vi "Create Table Refnum.vi"(0 "PDF Report":refnum<class "PDF Report Class.lvclass">, 1 "Table properties":T1={"Table position"=1, "SpacingBefore (points)"=12.0, "SpacingAfter (points)"=12.0} {"Table position" items=["LEFT", "CENTER", "RIGHT"]}, 5 "numColumns":i32, 9 "columnWidth [ ]":sgl[](array[numeric])=[0.0], 11 "error in (no error)":errorcluster, 12 "Repeat on each new page?":bool, 13 "HeaderRows":i32) -> (4 "PDF Report duplicate":refnum<class "PDF Report Class.lvclass">, 6 "columnWidth (points)":sgl[](array[numeric]), 8 "PdfP Table ref":refnum<k24>, 15 "error out":errorcluster)   [LabVIEW 2019]
doc: "<B>ENGLISH</B>\nCreates a table with the given <B>numColumns</B> and the given <B>columnWidth [ ]</B>.\n\n<B>FRANÇAIS</B>\nCréation d'un tableau avec pour nombre de colonnes <B>numColumns</B> et dont les largeurs sont spécifiées par <B>columnWidth [ ]</B>.\n\nVersion 2.0\nDeveloped by Jean-Marc Simard\nCopyright © 2012, Exaprom Inc.\nAll rights reserved.\nLicense: BSD\n\nWith iTextSharp 4.1.6 (http://itextsharp.sourceforge.net)\nunder Mozilla Public License Version 1.1\n(http://www.mozilla.org/MPL/MPL-1.1.html)"
uses:
  <userlib>/Exaprom PDF/LV Class/PDF Report Class/PDF Report Class.lvclass
  C:/Program Files/National Instruments/LabVIEW 2019/user.lib/Exaprom PDF/DLL/itextsharp.dll
  DLL/itextsharp.dll
  <userlib>/Exaprom PDF/Controls/Table Controls/Table properties.ctl
  <userlib>/Exaprom PDF/Controls/Table Controls/Table position.ctl
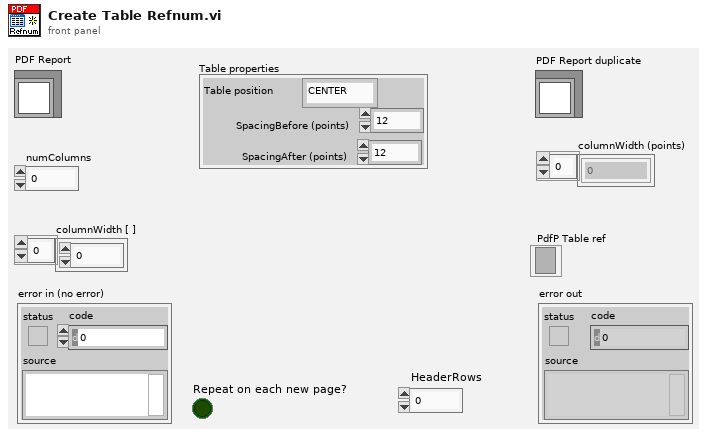
[diagram p1: front panel]
types:
  T1 = typedef "Table properties.ctl" = cluster{"Table position":T2, "SpacingBefore (points)":sgl, "SpacingAfter (points)":sgl}
  T2 = typedef "Table position.ctl" = i32
  T3 = typedef "Page dimensions.ctl" = cluster{"Start at page":i32, "Page Size":T4, "Orientation":T5, "widht":sgl, "height":sgl, "Margin left":sgl, "Margin right":sgl, "Margin top":sgl, "Margin bottom":sgl, "X0":sgl, "X1":sgl, "Y0":sgl, "Y1":sgl}
  T4 = typedef "Page size.ctl" = i32
  T5 = typedef "Page Orientation.ctl" = enum16{"Portrait", "Landscape"}
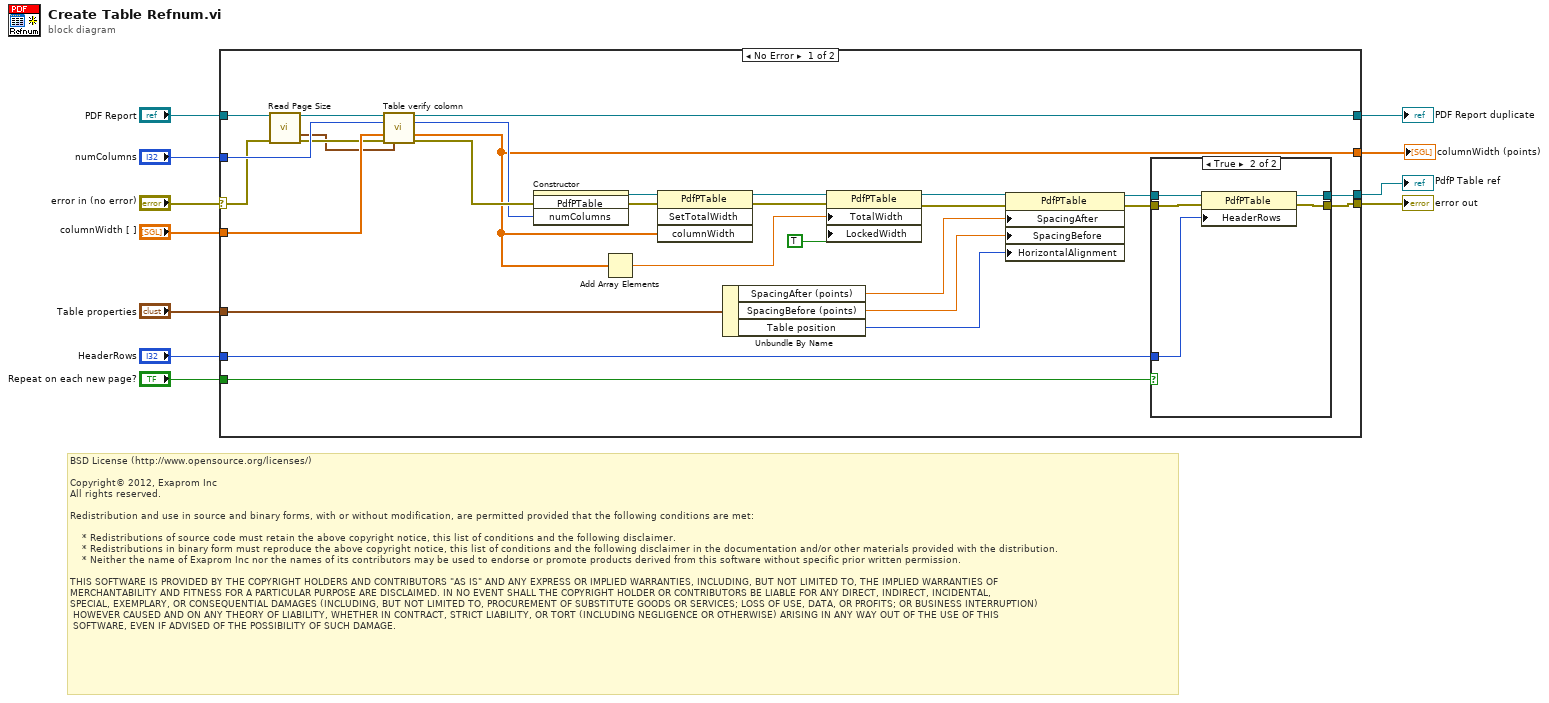
[diagram p0: block diagram]
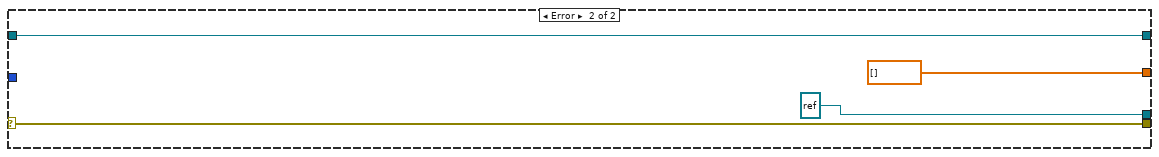
[diagram p3: hidden frame]
diagram:
  # "BSD License (http://www.opensource.org/licenses/)\n\nCopyright© 2012, Exaprom Inc\nAll rights reserved.\n\nRedistribution and use in source and binary forms, with or without modification, are permitted provided that the following conditions are met:\n\n    * Redistributions of source code must retain the above copyright notice, this list of conditions and the following disclaimer.\n    * Redistributions in binary form must reproduce the above copyright notice, this list of conditions and the following disclaimer in the documentation and/or other materials provided with the distribution.\n    * Neither the name of Exaprom Inc nor the names of its contributors may be used to endorse or promote products derived from this software without specific prior written permission.\n\nTHIS SOFTWARE IS PROVIDED BY THE COPYRIGHT HOLDERS AND CONTRIBUTORS \"AS IS\" AND ANY EXPRESS OR IMPLIED WARRANTIES, INCLUDING, BUT NOT LIMITED TO, THE IMPLIED WARRANTIES OF \nMERCHANTABILITY AND FITNESS FOR A PARTICULAR PURPOSE ARE DISCLAIMED. IN NO EVENT SHALL THE COPYRIGHT HOLDER OR CONTRIBUTORS BE LIABLE FOR ANY DIRECT, INDIRECT, INCIDENTAL,\nSPECIAL, EXEMPLARY, OR CONSEQUENTIAL DAMAGES (INCLUDING, BUT NOT LIMITED TO, PROCUREMENT OF SUBSTITUTE GOODS OR SERVICES; LOSS OF USE, DATA, OR PROFITS; OR BUSINESS INTERRUPTION)\n HOWEVER CAUSED AND ON ANY THEORY OF LIABILITY, WHETHER IN CONTRACT, STRICT LIABILITY, OR TORT (INCLUDING NEGLIGENCE OR OTHERWISE) ARISING IN ANY WAY OUT OF THE USE OF THIS\n SOFTWARE, EVEN IF ADVISED OF THE POSSIBILITY OF SUCH DAMAGE."
  n1 = case shown="No Error" "error in (no error)" {
    selector: "error in (no error)" -> [w18 w51]
    tunnel: "numColumns" -> [w31 _]
    tunnel: "columnWidth [ ]" -> [w32 _]
    tunnel: [w15 w51] -> w8
    tunnel: [w16 refnum<k24> refnum ("new reference")] -> w7
    tunnel: [w30 w49] -> w6
    tunnel: "PDF Report" -> [w28 w49]
    tunnel: "Table properties" -> [w23 _]
    tunnel: [w19 sgl[] [] ("columnWidth (points)")] -> w3
    tunnel: "Repeat on each new page?" -> [w13 _]
    tunnel: "HeaderRows" -> [w12 _]
    frame No Error {
      n2 = call <userlib>:"Read Page Size.vi"("PDF Report"=w28, "error in (no error)"=w18) -> ("PDF Report duplicate"=w29:refnum<class "PDF Report Class.lvclass">, "Page (points)"=w26:T3, "error out"=w27:errorcluster)  [unwired: 11 out]
      n3 = call <userlib>:"Table verify colomn.vi"("PDF Report"=w29, "numColumns"=w31, "columnWidth"=w32, "error in (no error)"=w27, "Pages dimensions"=w26) -> ("PDF Report duplicate"=w30:refnum<class "PDF Report Class.lvclass">, "numColumns duplicate"=w33:i32, "columnWidth (points)"=w19:sgl[], "error out"=w34:errorcluster)  [unwired: 7 out]
      n4 = constructor class="PdfPTable"(error in=w34, "numColumns"=w33) -> (reference out=w39:refnum<k24>, error out=w40:errorcluster)  [unwired: 2 in, 2 out]
      n5 = Add Array Elements(numeric array=w19) -> (sum=w35:sgl)
      n6 = invoke class="PdfPTable" method="SetTotalWidth"(reference=w39, error in=w40, "columnWidth"=w19) -> (reference out=w38:refnum<k24>, error out=w37:errorcluster)  [unwired: 1 in, 2 out]
      n7 = Unbundle By Name(w23) -> ("SpacingAfter (points)"=w22:sgl, "SpacingBefore (points)"=w21:sgl, "Table position"=w20:T2)
      n8 = property class="PdfPTable"(reference=w38, error in=w37, "TotalWidth"=w35, "LockedWidth"=TRUE) -> (reference out=w25:refnum<k24>, error out=w24:errorcluster)
      n9 = property class="PdfPTable"(reference=w25, error in=w24, "SpacingAfter"=w22, "SpacingBefore"=w21, "HorizontalAlignment"=w20) -> (reference out=w17:refnum<k24>, error out=w14:errorcluster)
      n10 = case shown="True" w13 {
        tunnel: w12 -> [_ w43]
        tunnel: w17 -> [w42 w47]
        tunnel: w14 -> [w41 w46]
        tunnel: [w42 w44] -> w16
        tunnel: [w41 w45] -> w15
        frame False {
        }
        frame True {
          n11 = property class="PdfPTable"(reference=w47, error in=w46, "HeaderRows"=w43) -> (reference out=w44:refnum<k24>, error out=w45:errorcluster)
        }
      }
    }
    frame Error {
    }
  }
  "error out" <- w8
  "PDF Report duplicate" <- w6
  "PdfP Table ref" <- w7
  "columnWidth (points)" <- w3
